vi "S_SKT_GLBL.vi"() -> ()   [LabVIEW 2016]
uses:
  D:/share/ProtoDUNE/LABVIEW/S_SKT_ADC_CTST/S_SKT_ADC_DLL/S_SKT_ADC_DLL/bin/Debug/S_SKT_ADC_DLL.dll
  S_SKT_ADC_DLL/S_SKT_ADC_DLL/bin/Debug/S_SKT_ADC_DLL.dll
panel:
  out "S_SKT_DLL":refnum<k24>
  out "UDP/I2C":bool=TRUE
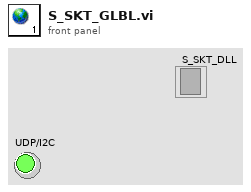
[diagram p1: front panel]
diagram:
